vi "VI HovaCAL KGN Test.vi"(5 "Set Values Cluster":T10(array[cluster])=[{"input concentration setpoint"=0.0, "output concentration setpoint"=0.0}, {"input concentration setpoint"=0.0, "output concentration setpoint"=0.0}, {"input concentration setpoint"=0.0, "output concentration setpoint"=0.0}, {"input concentration setpoint"=0.0, "output concentration setpoint"=0.0}, {"input concentration setpoint"=0.0, "output concentration setpoint"=0.0}] {"output concentration setpoint" format="%.2f"; "input concentration setpoint" format="%.2f"}, 6 "Stopp":bool, 8 "error in (no error)":errorcluster, 9 "MFC Cluster":T2 {"MFC Flow Cluster"."max flow" format="%.2f"; "MFC Flow Cluster"."min flow" format="%.2f"; "MFC Pump Temp Cluster"."Temp" items=["TmpCtrl0"]; "MFC Pump Temp Cluster"."Pump" items=["Pump0"]; "MFC Pump Temp Cluster"."MFC" items=["MFV0", "MFV1", "MFV2"]}, 10 "Input Cluster":T7 {"Flow Input Cluster"."total flow setpoint" format="%.2f"; "PumpMode-Cluster"."concentratio mode" items=["water", "reagent"]; "PumpMode-Cluster"."Reagent" items=["HCl", "HF", "NH3", "HG", "PPM", "ORGANIC"]; "PumpModeGeneral-Cluster"."dry mode" items=["wet", "dry"]; "PumpModeGeneral-Cluster"."control mode" items=["static", "pid"]; "Temperature" format="%.2f"}, 11 "Comm Cluster":T9={"serial port name"="COM3", "Comm Ports"=0, "Connect"=FALSE} {"Comm Ports" items=["COM4", "LPT1"]}) -> (0 "error out":errorcluster, 2 "Output Cluster":T8 {"PumpGeneral-Cluster"."dry mode" items=["wet", "dry"]; "PumpGeneral-Cluster"."control mode" items=["static", "pid"]; "Flow Output Cluster"."total flow" format="%.2f"; "Flow Output Cluster"."total flow setpoint" format="%.2f"; "Temp Cluster"."humidity" format="%.2f"; "Temp Cluster"."temp" format="%.2f"; "Temp Cluster"."temp SP" format="%.2f"; "PumpMode-Cluster"."concentratio mode" items=["water", "reagent"]; "PumpMode-Cluster"."Reagent" items=["HCl", "HF", "NH3", "HG", "PPM", "ORGANIC"]}, 3 "Actual Values Cluster":T11(array[cluster]) {"output concentration dry" format="%.2f"; "output concentration" format="%.2f"; "output concentration setpoint" format="%.2f"; "input concentration setpoint" format="%.2f"}, 4 "System Cluster":T1)   [LabVIEW 2020, in "Linearisierung v2.lvlib" / "Gasteiler.lvlib" / "HovaCAL_Interface.lvlib" / "KGN.lvlib"]
uses:
  KGN.lvlib
  Controls/Info Cluster.ctl
  Controls/Controls.lvlib
  set/set.lvlib
  GUI Get/KGN GUI Get.lvlib
  GUI Set/KGN GUI Set.lvlib
  Helper/Helper.lvlib
  Allgemein/allgemeine Sub-VIs.lvlib
  Controls/Reagent.ctl
  Controls/Pump Control Mode.ctl
  Controls/Pump Dry Mode.ctl
  Controls/Pump Concentration Mode.ctl
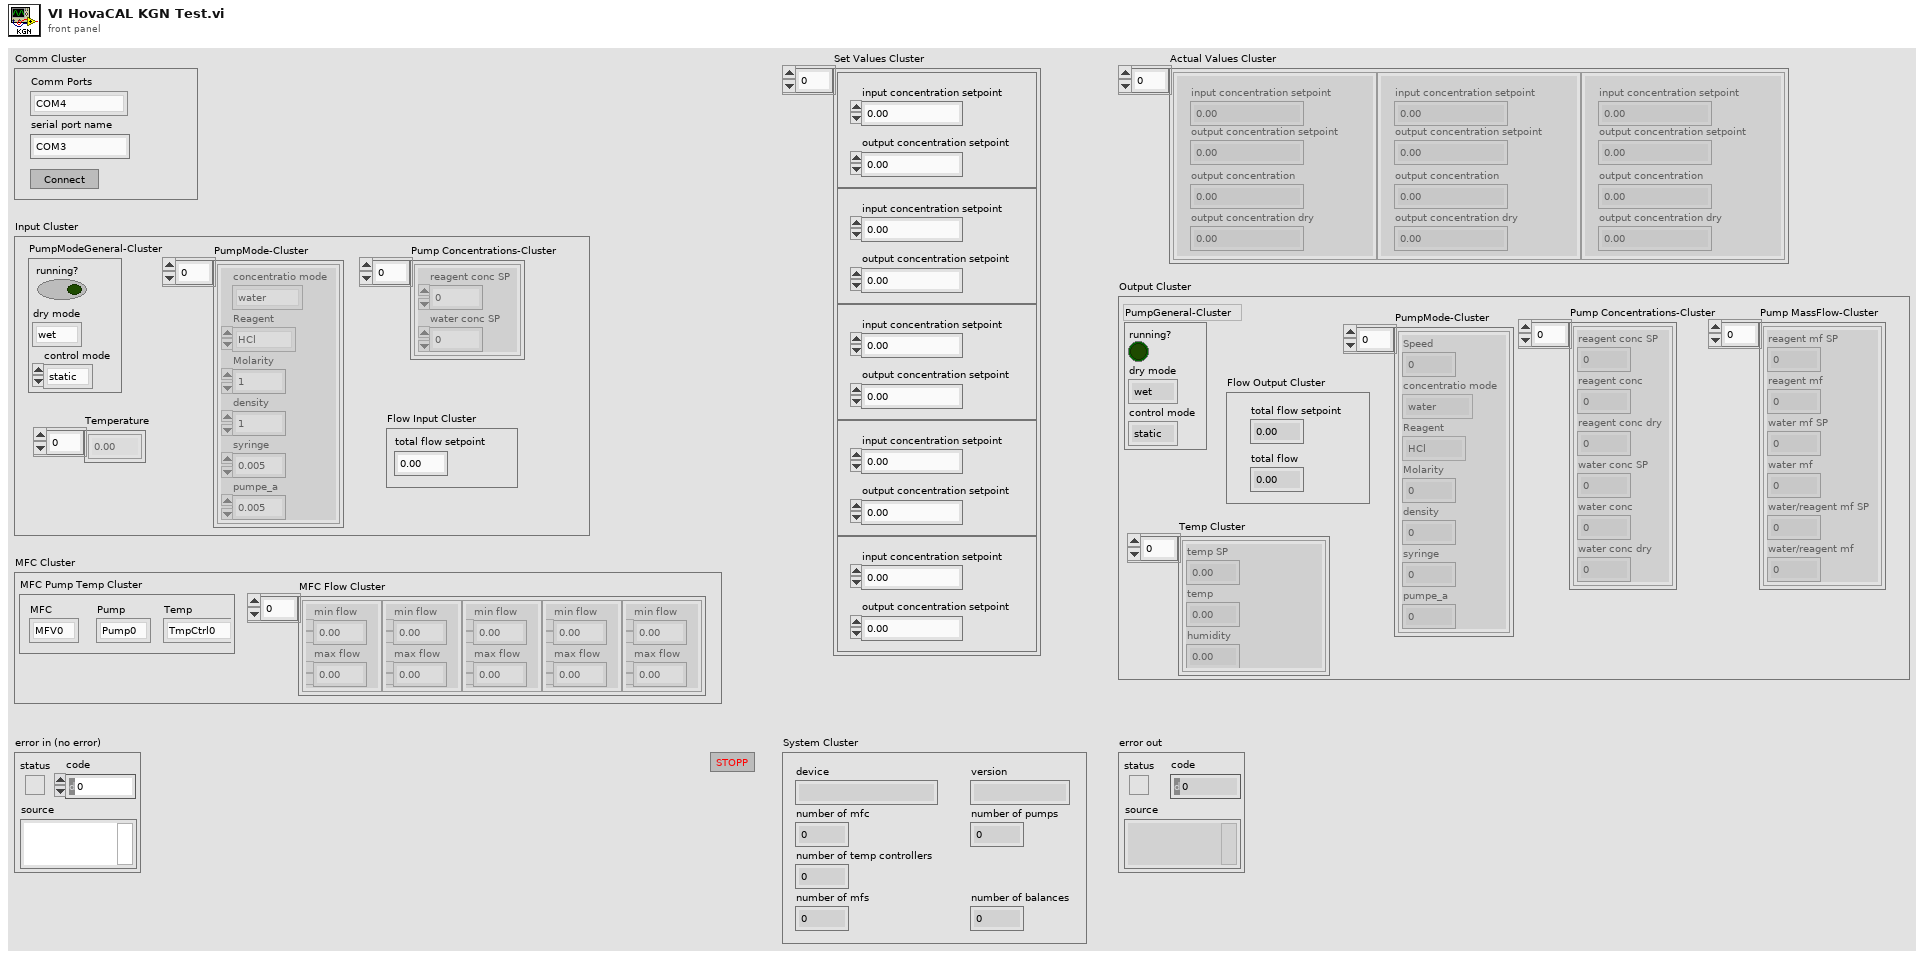
[diagram p1: front panel]
types:
  T1 = cluster{"device":string, "version":string, "number of mfc":i32, "number of pumps":i32, "number of temp controllers":i32, "number of mfs":i32, "number of balances":i32}
  T2 = cluster{"MFC Pump Temp Cluster":cluster{"MFC":u16, "Pump":u16, "Temp":u16}, "MFC Flow Cluster":cluster{"min flow":dbl, "max flow":dbl}[]}
  T3 = typedef "Linearisierung v2.lvlib/Gasteiler.lvlib/HovaCAL_Interface.lvlib/Controls.lvlib/Pump Dry Mode.ctl" = i32
  T4 = typedef "Linearisierung v2.lvlib/Gasteiler.lvlib/HovaCAL_Interface.lvlib/Controls.lvlib/Pump Control Mode.ctl" = u32
  T5 = typedef "Linearisierung v2.lvlib/Gasteiler.lvlib/HovaCAL_Interface.lvlib/Controls.lvlib/Pump Concentration Mode.ctl" = i32
  T6 = typedef "Linearisierung v2.lvlib/Gasteiler.lvlib/HovaCAL_Interface.lvlib/Controls.lvlib/Reagent.ctl" = i32
  T7 = cluster{"Temperature":dbl[], "PumpModeGeneral-Cluster":cluster{"running?":bool, "dry mode":T3, "control mode":T4}, "PumpMode-Cluster":cluster{"concentratio mode":T5, "Reagent":T6, "Molarity":dbl, "density":dbl, "syringe":dbl, "pumpe_a":dbl}[], "Flow Input Cluster":cluster{"total flow setpoint":dbl}, "Pump Concentrations-Cluster":cluster{"reagent conc SP":dbl, "water conc SP":dbl}[]}
  T8 = cluster{"Temp Cluster":cluster{"temp SP":dbl, "temp":dbl, "humidity":dbl}[], "PumpGeneral-Cluster":cluster{"running?":bool, "dry mode":T3, "control mode":T4}, "PumpMode-Cluster":cluster{"Speed":dbl, "concentratio mode":T5, "Reagent":T6, "Molarity":dbl, "density":dbl, "syringe":dbl, "pumpe_a":dbl}[], "Pump Concentrations-Cluster":cluster{"reagent conc SP":dbl, "reagent conc":dbl, "reagent conc dry":dbl, "water conc SP":dbl, "water conc":dbl, "water conc dry":dbl}[], "Flow Output Cluster":cluster{"total flow setpoint":dbl, "total flow":dbl}, "Pump MassFlow-Cluster":cluster{"reagent mf SP":dbl, "reagent mf":dbl, "water mf SP":dbl, "water mf":dbl, "water/reagent mf SP":dbl, "water/reagent mf":dbl}[]}
  T9 = cluster{"serial port name":string, "Comm Ports":u16, "Connect":bool}
  T10 = cluster{"input concentration setpoint":dbl, "output concentration setpoint":dbl}[]
  T11 = cluster{"input concentration setpoint":dbl, "output concentration setpoint":dbl, "output concentration":dbl, "output concentration dry":dbl}[]
  T12 = enum8{"Enabled", "Disabled", "Disabled and Grayed Out"}
  T13 = cluster{"MFC Pump Temp Cluster":refnum<vi>, "Set Values Cluster":refnum<vi>, "Input Cluster":refnum<vi>}
  T14 = typedef "Linearisierung v2.lvlib/Gasteiler.lvlib/HovaCAL_Interface.lvlib/Controls.lvlib/Info Cluster.ctl" = cluster{"device":string, "version":string, "number of mfc":i32, "number of pumps":i32, "number of temp controllers":i32, "number of mfs":i32, "number of balances":i32}
  T15 = cluster{"Input Concentrations (Ausgang)":cluster{"input concentration setpoint":dbl, "output concentration setpoint":dbl, "output concentration":dbl, "output concentration dry":dbl}[], "Cluster":cluster{"Temp Cluster":cluster{"temp SP":dbl, "temp":dbl, "humidity":dbl}[], "PumpModeGeneral-Cluster":cluster{"running?":bool, "dry mode":T3, "control mode":T4}, "PumpMode-Cluster":cluster{"Speed":dbl, "concentratio mode":T5, "Reagent":T6, "Molarity":dbl, "density":dbl, "syringe":dbl, "pumpe_a":dbl}[], "Pump Concentrations-Cluster":cluster{"reagent conc SP":dbl, "reagent conc":dbl, "reagent conc dry":dbl, "water conc SP":dbl, "water conc":dbl, "water conc dry":dbl}[], "Flow Output Cluster (Ausgang)":cluster{"total flow setpoint":dbl, "total flow":dbl}, "Pump MassFlow-Cluster":cluster{"reagent mf SP":dbl, "reagent mf":dbl, "water mf SP":dbl, "water mf":dbl, "water/reagent mf SP":dbl, "water/reagent mf":dbl}[]}}
  T16 = cluster{"Temperature":dbl[], "PumpModeGeneral-Cluster":cluster{"running?":bool, "dry mode":T3, "control mode":T4}, "PumpMode-Cluster":cluster{"concentratio mode":T5, "Reagent":T6, "Molarity":dbl, "density":dbl, "syringe":dbl, "pump_a":dbl}[], "Flow Input Cluster":cluster{"total flow setpoint":dbl}, "Pump Concentrations-Cluster":cluster{"reagent conc SP":dbl, "water conc SP":dbl}[]}
  T17 = cluster{"Temp Cluster":cluster{"temp SP":dbl, "temp":dbl, "humidity":dbl}[], "PumpModeGeneral-Cluster":cluster{"running?":bool, "dry mode":T3, "control mode":T4}, "PumpMode-Cluster":cluster{"Speed":dbl, "concentratio mode":T5, "Reagent":T6, "Molarity":dbl, "density":dbl, "syringe":dbl, "pumpe_a":dbl}[], "Pump Concentrations-Cluster":cluster{"reagent conc SP":dbl, "reagent conc":dbl, "reagent conc dry":dbl, "water conc SP":dbl, "water conc":dbl, "water conc dry":dbl}[], "Flow Output Cluster (Ausgang)":cluster{"total flow setpoint":dbl, "total flow":dbl}, "Pump MassFlow-Cluster":cluster{"reagent mf SP":dbl, "reagent mf":dbl, "water mf SP":dbl, "water mf":dbl, "water/reagent mf SP":dbl, "water/reagent mf":dbl}[]}
  T18 = cluster{"running?":bool, "dry mode":T3, "control mode":T4}
  T19 = cluster{"reagent conc SP":dbl, "water conc SP":dbl}[]
  T20 = cluster{"concentratio mode":T5, "Reagent":T6, "Molarity":dbl, "density":dbl, "syringe":dbl, "pumpe_a":dbl}[]
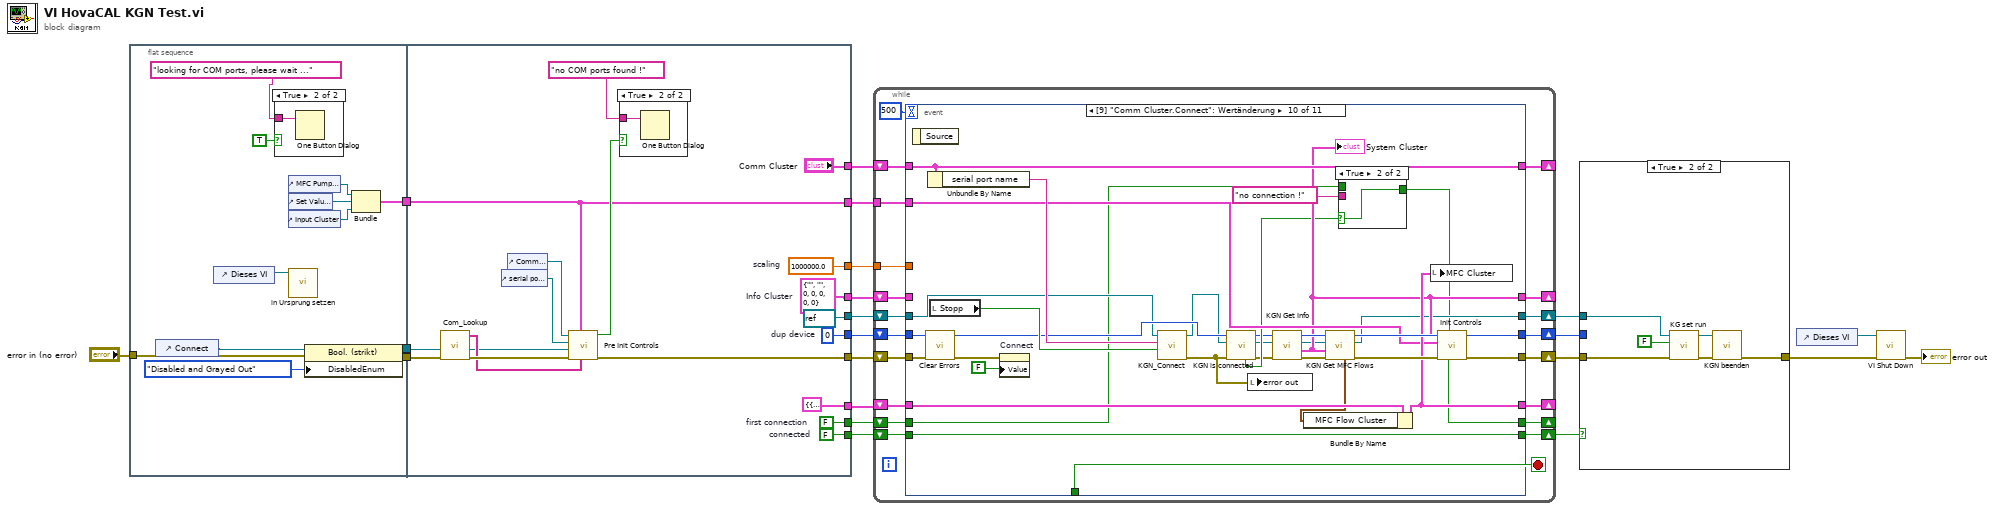
[diagram p0: block diagram]
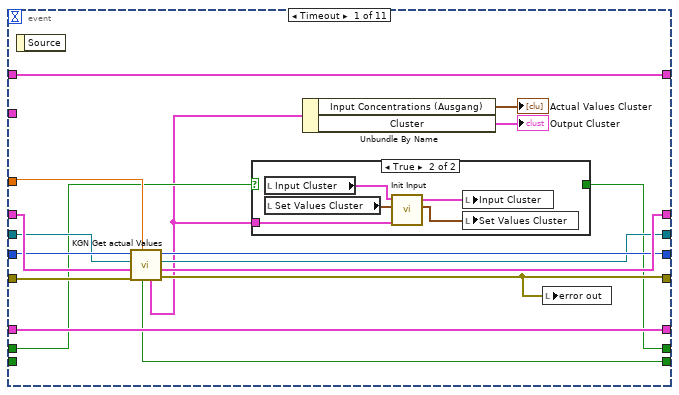
[diagram p5: hidden frame]
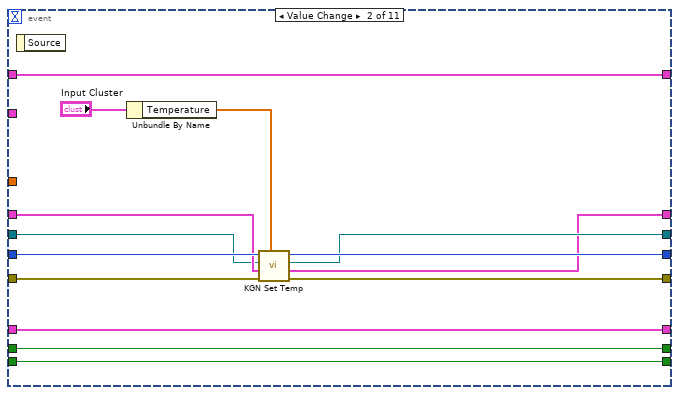
[diagram p7: hidden frame]
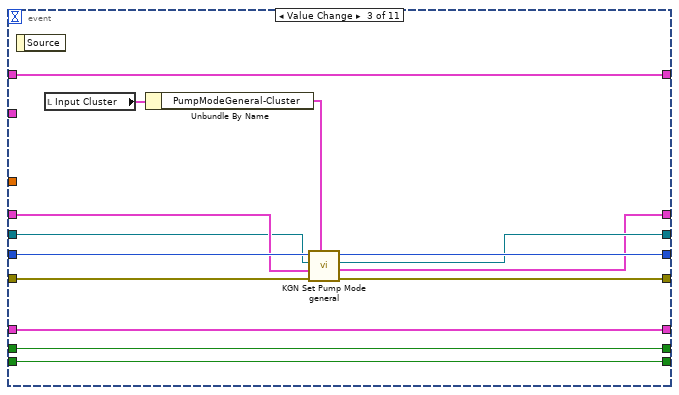
[diagram p8: hidden frame]
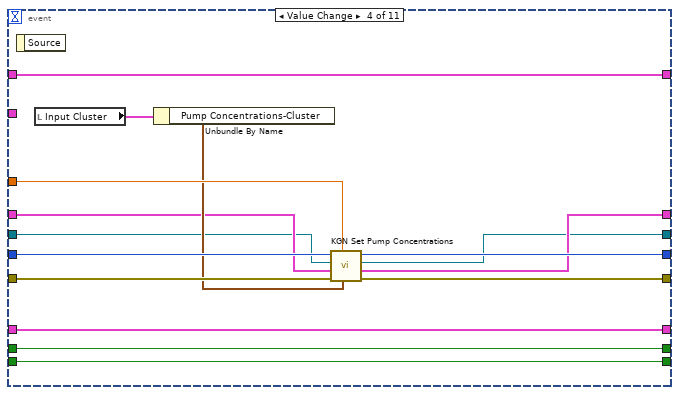
[diagram p9: hidden frame]
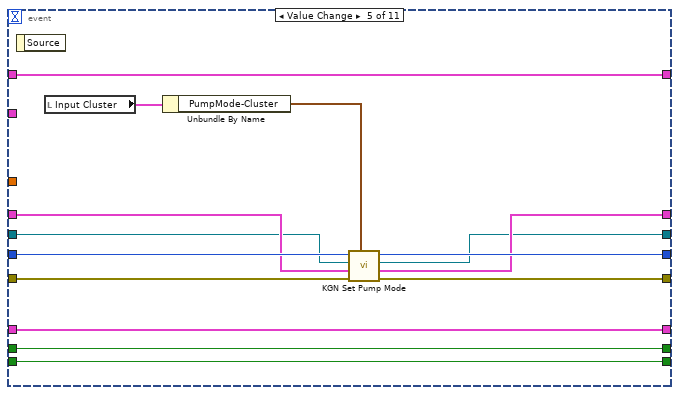
[diagram p10: hidden frame]
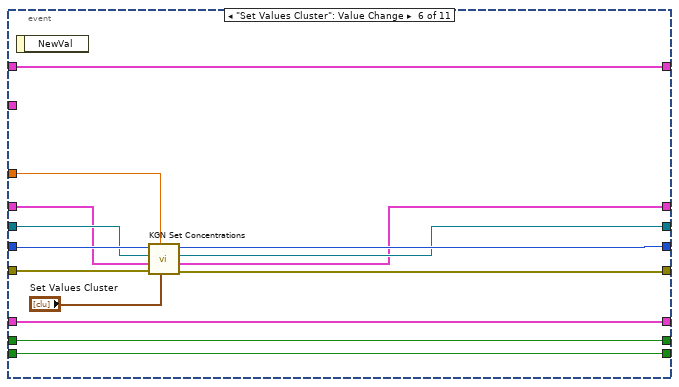
[diagram p11: hidden frame]
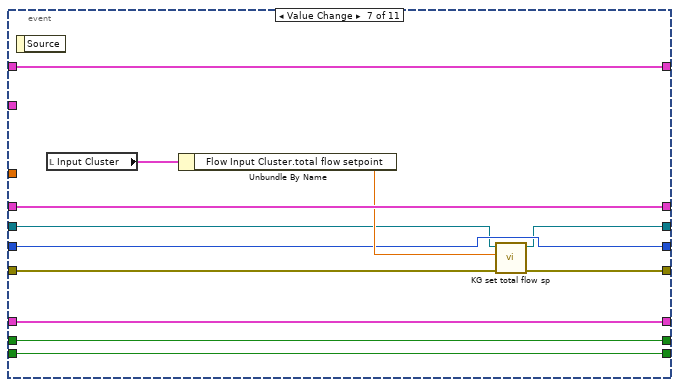
[diagram p12: hidden frame]
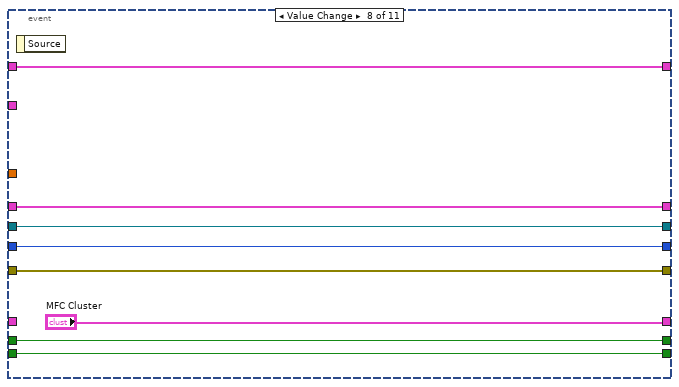
[diagram p13: hidden frame]
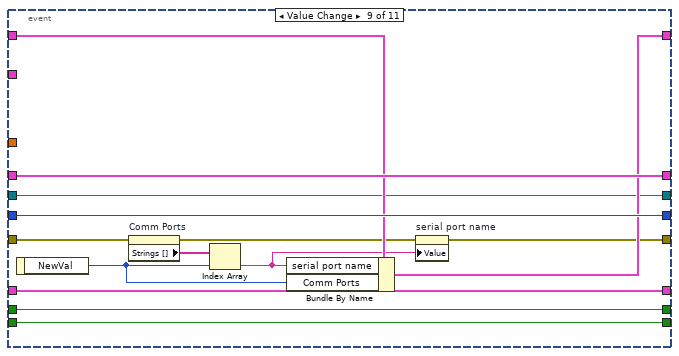
[diagram p14: hidden frame]
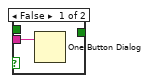
[diagram p15: hidden frame]
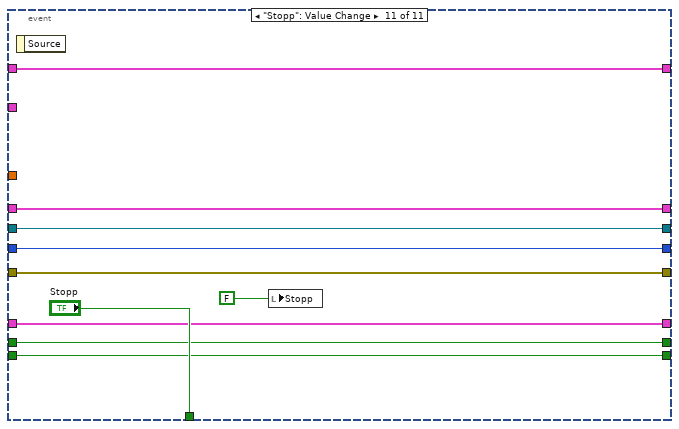
[diagram p16: hidden frame]
diagram:
  n1 = flat-sequence {
    tunnel: "error in (no error)" -> [w25]
    tunnel: [w31] -> w14
    tunnel: [w28] -> w13
    tunnel: [w21] -> w3
    tunnel: [w46] -> w17
    tunnel: [w49] -> w16
    tunnel: ["Comm Cluster"] -> w15
    tunnel: w14 -> [w50]
    tunnel: w13 -> [w36]
    tunnel: [w44] -> w12
    tunnel: [w43] -> w11
    tunnel: [T2 {"MFC Pump Temp Cluster"={"MFC"=0, "Pump"=0, "Temp"=0}, "MFC Flow Cluster"=[]} ("MFC Cluster")] -> w10
    tunnel: [refnum<visa-resource-name> refnum ("VISA-Ressourcenname out")] -> w8
    tunnel: [w41] -> w7
    tunnel: [w40] -> w5
    tunnel: w3 -> [w35]
    tunnel: [w35] -> w2
    frame #0 {
      n2 = control-ref of="Connect"() -> (w26:refnum<vi>)
      n3 = control-ref of="Dieses VI"() -> (w27:refnum<vi>)
      n4 = case shown="True" TRUE {
        tunnel: "looking for COM ports, please wait ..." -> [_ w33]
        frame False {
        }
        frame True {
          n5 = One Button Dialog(message=w33) -> ()  [unwired: 1 in, 1 out]
        }
      }
      n6 = control-ref of="MFC Pump Temp Cluster"() -> (w23:refnum<vi>)
      n7 = control-ref of="Set Values Cluster"() -> (w22:refnum<vi>)
      n8 = control-ref of="Input Cluster"() -> (w24:refnum<vi>)
      n9 = call "in Ursprung setzen.vi"("VI Referenz"=w27) -> ()  [unwired: 11 in]
      n10 = property class="Bool. (strikt)"(reference=w26, error in=w25, "DisabledEnum"=T12."Disabled and Grayed Out" ("Deaktiviert")) -> (reference out=w28:refnum<vi>, error out=w31:errorcluster)
      n11 = Bundle("MFC Pump Temp Cluster"=w23, "Set Values Cluster"=w22, "Input Cluster"=w24) -> (w21:T13)  [unwired: 1 in]
    }
    frame #1 {
      w40 = FALSE  # connected
      w41 = FALSE  # first connection
      w43 = T14 {"device"="", "version"="", "number of mfc"=0, "number of pumps"=0, "number of temp controllers"=0, "number of mfs"=0, "number of balances"=0}  # Info Cluster
      w44 = u32 0  # dup device
      w49 = 1000000.0  # scaling
      n12 = call "Com_Lookup.vi"("Fehler (Eingang, kein Fehler)"=w50) -> ("Fehler (Ausgang)"=w51:errorcluster, "find list"=w39:string[])  [unwired: 9 in]
      n13 = control-ref of="serial port name"() -> (w37:refnum<vi>)
      n14 = control-ref of="Comm Ports"() -> (w38:refnum<vi>)
      n15 = call "Pre Init Controls.vi"("find list"=w39, "Cluster Refernz Cluster"=w35, "Fehler (Eingang, kein Fehler)"=w51, "Connect Referenz"=w36, "Str Referenz"=w37, "Ring (Eingang)"=w38) -> ("Fehler (Ausgang)"=w46:errorcluster, "empty?"=w45:bool)  [unwired: 4 in]
      n16 = case shown="True" w45 {
        tunnel: "no COM ports found !" -> [_ w52]
        frame False {
        }
        frame True {
          n17 = One Button Dialog(message=w52) -> ()  [unwired: 1 in, 1 out]
        }
      }
    }
  }
  n18 = while {
    shift-right: [w69] -> w20
    shift-left: w12 -> [w70]
    shift-right: [w67] -> w19
    shift-left: w17 -> [w68]
    shift-right: [w66] -> _
    shift-left: w10 -> [w65]
    tunnel: w16 -> [w63]
    shift-right: [w62] -> _
    shift-left: w11 -> [w64]
    shift-right: [w60] -> _
    shift-left: w15 -> [w61]
    tunnel: w2 -> [w59]
    shift-right: [w58] -> w9
    shift-left: w8 -> [w57]
    shift-right: [w55] -> _
    shift-left: w7 -> [w56]
    shift-right: [w54] -> w4
    shift-left: w5 -> [w53]
    stop <- w71 stop-if-true
    n19 = event shown="[9] \"Comm Cluster.Connect\": Wertänderung" {
      selector: _ -> [_ _ _ _ _ _ _ _ _ _ _]
      dyn-events: _ -> [_ _ _ _ _ _ _ _ _ _ _]
      timeout: 500 -> [_ _ _ _ _ _ _ _ _ _ _]
      tunnel: [_ _ _ _ _ _ _ _ _ _ "Stopp"] -> w71
      tunnel: w70 -> [w81 w107 w120 w136 w149 w165 w174 w186 w200 w226 w242]
      tunnel: [w79 w106 w117 w135 w148 w162 w174 w186 w200 w223 w242] -> w69
      tunnel: w68 -> [w89 w105 w119 w133 w146 w161 w173 w185 w194 w225 w241]
      tunnel: [w77 w104 w118 w134 w147 w160 w172 w185 w190 w213 w241] -> w67
      tunnel: [w88 w109 w123 w138 w152 w163 w178 "MFC Cluster" w199 w221 w240] -> w66
      tunnel: w65 -> [w88 w109 w123 w138 w152 w163 w178 _ w199 w231 w240]
      tunnel: w63 -> [w82 _ _ w132 _ w166 _ _ _ _ _]
      tunnel: w64 -> [w86 w102 w115 w129 w145 w156 w177 w184 w197 _ w238]
      tunnel: [w83 w98 w112 w128 w144 w155 w177 w184 w197 w216 w238] -> w62
      tunnel: w61 -> [w87 w108 w122 w137 w151 w164 w176 w183 w196 w228 w237]
      tunnel: [w87 w108 w122 w137 w151 w164 w176 w183 w195 w228 w237] -> w60
      tunnel: w59 -> [_ _ _ _ _ _ _ _ _ w220 _]
      tunnel: [w78 w99 w113 w126 w142 w157 w170 w181 w189 w214 w236] -> w58
      tunnel: w57 -> [w80 w100 w114 w127 w143 w158 w169 w181 w189 w219 w236]
      tunnel: w56 -> [w76 w97 w111 w125 w140 w154 w168 w180 w188 w205 w235]
      tunnel: [w75 w97 w111 w125 w140 w154 w168 w180 w188 w202 w235] -> w55
      tunnel: [w73 w96 w110 w124 w139 w153 w167 w179 w187 w204 w234] -> w54
      tunnel: w53 -> [_ w96 w110 w124 w139 w153 w167 w179 w187 w204 w234]
      event Timeout {
        n20 = event-data() -> ()  [unwired: 1 in, 1 out]
        n21 = call "KGN Get actual Values.vi"("scaling"=w82, "Fehler (Eingang, kein Fehler)"=w89, "Info Cluster"=w86, "VISA-Referenz (Eingang)"=w80, "device (Eingang)"=w81) -> ("Fehler (Ausgang)"=w77:errorcluster, "Info Cluster out"=w83:T14, "VISA-Referenz (Ausgang)"=w78:refnum<visa-resource-name>, "dup device (Ausgang)"=w79:u32, "actual Values Cluster"=w74:T15, "connected"=w73:bool)  [unwired: 1 in]
        n22 = case shown="True" w76 {
          selector: w76 -> [w90 _]
          tunnel: [w90 _] -> w75
          tunnel: w74 -> [_ w93]
          frame False {
          }
          frame True {
            n23 = local read "Input Cluster"() -> (w95:T7)
            n24 = local read "Set Values Cluster"() -> (w91:T10)
            n25 = call "Init Input.vi"("actual Values Cluster"=w93, "Set Values Cluster (Eingang)"=w91, "Input Cluster (Eingang)"=w95) -> ("Set Values Cluster (Ausgang)"=w92:T10, "Input Cluster (Ausgang)"=w94:T16)  [unwired: 7 in]
            n26 = local write "Input Cluster"(w94) -> ()
            n27 = local write "Set Values Cluster"(w92) -> ()
          }
        }
        n28 = Unbundle By Name(w74) -> ("Input Concentrations (Ausgang)"=→"Actual Values Cluster":T11, "Cluster"=→"Output Cluster":T17)
        n29 = local write "error out"(w77) -> ()
      }
      event "Input Cluster.Temperature": Value Change {
        n30 = event-data() -> ()  [unwired: 1 in, 1 out]
        n31 = Unbundle By Name("Input Cluster") -> ("Temperature"=w101:dbl[])
        n32 = call "KGN Set Temp.vi"("Temperature"=w101, "Fehler (Eingang, kein Fehler)"=w105, "Info Cluster"=w102, "VISA-Referenz (Eingang)"=w100, "device (Eingang)"=w107) -> ("Fehler (Ausgang)"=w104:errorcluster, "Info Cluster out"=w98:T14, "VISA-Referenz (Ausgang)"=w99:refnum<visa-resource-name>, "dup device (Ausgang)"=w106:u32)  [unwired: 3 in]
      }
      event "Input Cluster.PumpModeGeneral-Cluster": Value Change {
        n33 = event-data() -> ()  [unwired: 1 in, 1 out]
        n34 = local read "Input Cluster"() -> (w121:T7)
        n35 = Unbundle By Name(w121) -> ("PumpModeGeneral-Cluster"=w116:T18)
        n36 = call "KGN Set Pump Mode general.vi"("PumpModeGeneral-Cluster"=w116, "Fehler (Eingang, kein Fehler)"=w119, "Info Cluster"=w115, "VISA-Referenz (Eingang)"=w114, "device (Eingang)"=w120) -> ("Fehler (Ausgang)"=w118:errorcluster, "Info Cluster out"=w112:T14, "VISA-Referenz (Ausgang)"=w113:refnum<visa-resource-name>, "dup device (Ausgang)"=w117:u32)  [unwired: 3 in]
      }
      event "Input Cluster.Pump Concentrations-Cluster": Value Change {
        n37 = event-data() -> ()  [unwired: 1 in, 1 out]
        n38 = local read "Input Cluster"() -> (w131:T7)
        n39 = Unbundle By Name(w131) -> ("Pump Concentrations-Cluster"=w130:T19)
        n40 = call "KGN Set Pump Concentrations.vi"("Pump Concentrations-Cluster"=w130, "scaling"=w132, "Fehler (Eingang, kein Fehler)"=w133, "Info Cluster"=w129, "VISA-Referenz (Eingang)"=w127, "device (Eingang)"=w136) -> ("Fehler (Ausgang)"=w134:errorcluster, "Info Cluster out"=w128:T14, "VISA-Referenz (Ausgang)"=w126:refnum<visa-resource-name>, "dup device (Ausgang)"=w135:u32)  [unwired: 2 in]
      }
      event "Input Cluster.PumpMode-Cluster": Value Change {
        n41 = event-data() -> ()  [unwired: 1 in, 1 out]
        n42 = local read "Input Cluster"() -> (w150:T7)
        n43 = Unbundle By Name(w150) -> ("PumpMode-Cluster"=w141:T20)
        n44 = call "KGN Set Pump Mode.vi"("PumpMode-Cluster"=w141, "Fehler (Eingang, kein Fehler)"=w146, "Info Cluster"=w145, "VISA-Referenz (Eingang)"=w143, "device (Eingang)"=w149) -> ("Fehler (Ausgang)"=w147:errorcluster, "Info Cluster out"=w144:T14, "VISA-Referenz (Ausgang)"=w142:refnum<visa-resource-name>, "dup device (Ausgang)"=w148:u32)  [unwired: 3 in]
      }
      event "Set Values Cluster": Value Change {
        n45 = event-data() -> ()  [unwired: 1 in, 1 out]
        n46 = call "KGN Set Concentrations.vi"("Set Values Cluster"="Set Values Cluster", "scaling"=w166, "Fehler (Eingang, kein Fehler)"=w161, "Info Cluster"=w156, "VISA-Referenz (Eingang)"=w158, "device (Eingang)"=w165) -> ("Fehler (Ausgang)"=w160:errorcluster, "Info Cluster out"=w155:T14, "VISA-Referenz (Ausgang)"=w157:refnum<visa-resource-name>, "dup device (Ausgang)"=w162:u32)  [unwired: 2 in]
      }
      event "Input Cluster.Flow Input Cluster": Value Change {
        n47 = event-data() -> ()  [unwired: 1 in, 1 out]
        n48 = local read "Input Cluster"() -> (w171:T7)
        n49 = Unbundle By Name(w171) -> ("Flow Input Cluster.total flow setpoint"=w175:dbl)
        n50 = call "KG set total flow sp.vi"("Fehler (Eingang, kein Fehler)"=w173, "total flow setpoint"=w175, "VISA-Ressourcenname"=w169) -> ("Fehler (Ausgang)"=w172:errorcluster, "VISA-Ressourcenname (Ausgang)"=w170:refnum<visa-resource-name>)  [unwired: 7 in]
      }
      event "MFC Cluster.MFC Pump Temp Cluster": Value Change {
        n51 = event-data() -> ()  [unwired: 1 in, 1 out]
      }
      event "Comm Cluster.Comm Ports": Value Change {
        n52 = event-data() -> ("NewVal"=w193:u16)  [unwired: 1 in]
        n53 = property on="Comm Ports" class="Ring (strikt)"(error in=w194) -> (error out=w192:errorcluster, "Strings []"=w198:string[])  [unwired: 1 in, 1 out]
        n54 = Index Array(array=w198, index=w193) -> (element=w191:string)
        n55 = Bundle By Name(cluster=w196, "serial port name"=w191, "Comm Ports"=w193) -> (w195:T9)
        n56 = property on="serial port name" class="Str"(error in=w192, "Value"=w191) -> (error out=w190:errorcluster)  [unwired: 1 in, 1 out]
      }
      event "Comm Cluster.Connect": Value Change {
        n57 = event-data() -> ()  [unwired: 1 in, 1 out]
        n58 = call <vilib>:"Clear Errors.vi"("error in (no error)"=w225) -> ("error out"=w212:errorcluster)  [unwired: 5 in, 1 out]
        n59 = Unbundle By Name(w228) -> ("serial port name"=w229:string)
        n60 = local read "Stopp"() -> (w230:bool)
        n61 = property on="Connect" class="Bool. (strikt)"(error in=w212, "Value"=FALSE ("Wert")) -> ()  [unwired: 1 in, 2 out]
        n62 = call "KGN_Connect.vi"("Stopp"=w230, "serial port name"=w229, "VISA-Ressourcenname"=w219) -> ("Fehler (Ausgang)"=w209:errorcluster, "VISA-Ressourcenname (Ausgang)"=w211:refnum<visa-resource-name>)  [unwired: 5 in, 2 out]
        n63 = call "KGN is connected.vi"("Fehler (Eingang, kein Fehler)"=w209, "VISA-Ressourcenname"=w211, "device"=w226) -> ("Fehler (Ausgang)"=w207:errorcluster, "VISA-Ressourcenname out"=w208:refnum<visa-resource-name>, "dup device out"=w206:u32, "Boolesch"=w210:bool)  [unwired: 5 in]
        n64 = local write "error out"(w209) -> ()
        n65 = call "KGN Get Info.vi"("Fehler (Eingang, kein Fehler)"=w207, "VISA-Ressourcenname"=w208, "device"=w206) -> ("Fehler (Ausgang)"=w217:errorcluster, "System Cluster"=w216:T14, "VISA-Ressourcenname out"=w215:refnum<visa-resource-name>, "dup device"=w218:u32)  [unwired: 5 in]
        "System Cluster" <- w216
        n66 = call "KGN Get MFC Flows.vi"("Fehler (Eingang, kein Fehler)"=w217, "Info Cluster"=w216, "VISA-Ressourcenname"=w215, "device (Eingang)"=w218) -> ("Fehler (Ausgang)"=w222:errorcluster, "VISA-Ressourcenname out"=w214:refnum<visa-resource-name>, "dup device (Ausgang)"=w223:u32, "MFC Flow Cluster"=w201:cluster{"min flow":dbl, "max flow":dbl}[])  [unwired: 3 in, 1 out]
        n67 = Bundle By Name(cluster=w231, "MFC Flow Cluster"=w201) -> (w221:T2)
        n68 = case shown="True" w210 {
          selector: w210 -> [_ w233]
          tunnel: "no connection !" -> [w232 _]
          tunnel: w205 -> [_ _]
          tunnel: [_ w233] -> w203
          frame False {
            n69 = One Button Dialog(message=w232) -> ()  [unwired: 1 in, 1 out]
          }
          frame True {
          }
        }
        n70 = local write "MFC Cluster"(w221) -> ()
        n71 = call "Init Controls.vi"("connected"=w203, "Fehler (Eingang, kein Fehler)"=w222, "Cluster Refernz Cluster"=w220, "Info Cluster"=w216) -> ("Fehler (Ausgang)"=w213:errorcluster, "connected out"=w202:bool)  [unwired: 6 in]
      }
      event "Stopp": Value Change {
        n72 = event-data() -> ()  [unwired: 1 in, 1 out]
        n73 = local write "Stopp"(FALSE ("Stopp")) -> ()
      }
    }
  }
  n74 = case shown="True" w4 {
    tunnel: w20 -> [_ _]
    tunnel: w19 -> [w244 w250]
    tunnel: w9 -> [_ w249]
    tunnel: [w244 w248] -> w1
    frame False {
    }
    frame True {
      n75 = call "KG set run.vi"("Fehler (Eingang, kein Fehler)"=w250, "run"=FALSE, "VISA-Ressourcenname"=w249) -> ("Fehler (Ausgang)"=w245:errorcluster, "VISA-Ressourcenname (Ausgang)"=w246:refnum<visa-resource-name>)  [unwired: 7 in]
      n76 = call "KGN beenden.vi"("Fehler (Eingang, kein Fehler)"=w245, "VISA-Ressourcenname"=w246) -> ("Fehler (Ausgang)"=w248:errorcluster)  [unwired: 8 in, 1 out]
    }
  }
  "error out" <- w1
  n77 = control-ref of="Dieses VI"() -> (w6:refnum<vi>)
  n78 = call "VI Shut Down.vi"("VI Referenz"=w6) -> ()  [unwired: 11 in]
